vi "PmodACLOpen.vi"(7 "I2C Channel (0)":u8, 8 "Error In":errorcluster, 9 "Resolution":enum16{"2g", "4g", "8g", "16g"}(ring), 10 "ADXL345 Address":T1, 11 "LINX Resource":T2) -> (0 "Error Out":errorcluster, 1 "Resolution":enum16{"2g", "4g", "8g", "16g"}(ring), 3 "LINX Resource":T2)   [LabVIEW 2011, in "LMH-LINX.lvlib"]
doc: "Initialize the ADXL345 and bring it out of sleep mode."
uses:
  LMH-LINX.lvlib
  Private/Type Defs/LINX Ref.ctl
  Private/Type Defs/Platform.ctl
  Private/Type Defs/Interface.ctl
  Private/Device/Type Defs/LINX Device Config.ctl
  Private/Device/Type Defs/TCP Config.ctl
  Private/Device/Type Defs/Channels.ctl
  Accelerometer/ADXL345/Address.ctl
  Private/Device/Device.lvlib
  Accelerometer/ADXL345/ADXL345.lvlib
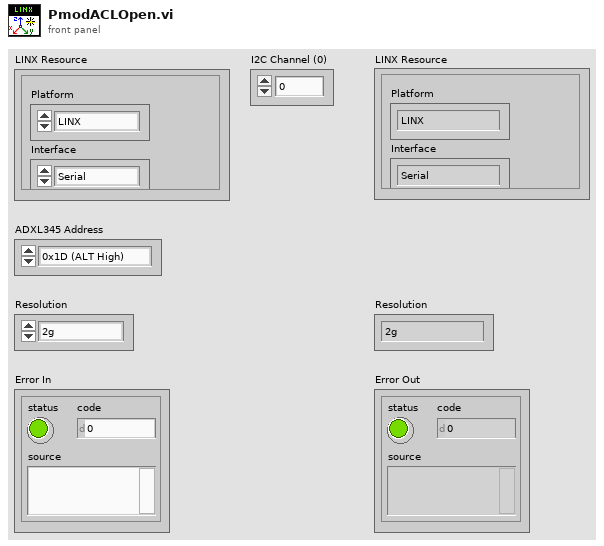
[diagram p1: front panel]
types:
  T1 = typedef "LMH-LINX.lvlib/ADXL345.lvlib/Address.ctl" = enum16{"0x1D (ALT High)", "0x53 (ALT Low)"}
  T2 = typedef "LMH-LINX.lvlib/LINX Ref.ctl" = cluster{"Platform":T3, "Interface":T4, "LINX Device Config":T5}
  T3 = typedef "LMH-LINX.lvlib/Platform.ctl" = enum16{"LINX", "myRIO"}
  T4 = typedef "LMH-LINX.lvlib/Interface.ctl" = enum16{"Serial", "TCP"}
  T5 = typedef "LMH-LINX.lvlib/Device.lvlib/LINX Device Config.ctl" = cluster{"Interface":T4, "COM Port":refnum<visa-resource-name>, "TCP Configuration":T6, "Device Family":u8, "Device ID":u8, "Device Name":string, "TCP Ref":refnum<k5>, "Channels":T7}
  T6 = typedef "LMH-LINX.lvlib/Device.lvlib/TCP Config.ctl" = cluster{"IP Address":string, "Port":u16}
  T7 = typedef "LMH-LINX.lvlib/Channels.ctl" = cluster{"DI":u8[], "DO":u8[], "AI":u8[], "AO":u8[], "PWM":u8[], "QE":u8[], "UART":u8[], "I2C 2":u8[], "SPI":u8[], "CAN":u8[], "Servo":u8[], "AI Ref (V)":dbl, "AO Ref (V)":dbl, "AO Resolution (Bits)":u8}
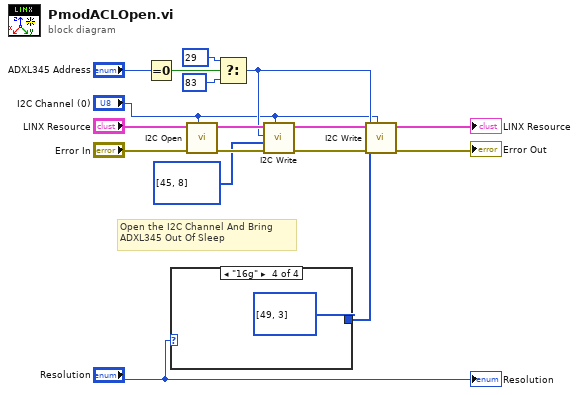
[diagram p0: block diagram]
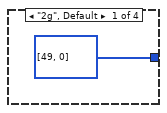
[diagram p2: hidden frame]
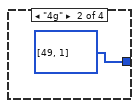
[diagram p3: hidden frame]
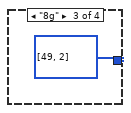
[diagram p4: hidden frame]
diagram:
  # "Open the I2C Channel And Bring \nADXL345 Out Of Sleep"
  n1 = Equal To 0?(x="ADXL345 Address") -> (x = 0?=w13:bool)
  n2 = case shown="\"16g\"" "Resolution" {
    tunnel: [u8[] [49, 0] ("Data") u8[] [49, 1] ("Data") u8[] [49, 2] ("Data") u8[] [49, 3] ("Data")] -> w7
    frame "2g", Default {
    }
    frame "4g" {
    }
    frame "8g" {
    }
    frame "16g" {
    }
  }
  n3 = call "I2C Open.vi"("I2C Channel (0)"="I2C Channel (0)", "Error In"="Error In", "LINX Resource"="LINX Resource") -> ("Error Out"=w16:errorcluster, "LINX Resource"=w17:T2)  [unwired: 7 in]
  n4 = Select(t=u8 29 ("I2C Slave Address (0)"), s=w13, f=u8 83 ("I2C Slave Address (0)")) -> (s? t:f=w2:u8)
  n5 = call "I2C Write.vi"("I2C Channel"="I2C Channel (0)", "Error In"=w16, "Data"=u8[] [45, 8], "I2C Slave Address (0)"=w2, "LINX Resource"=w17) -> ("Error Out"=w4:errorcluster, "LINX Resource"=w6:T2)  [unwired: 5 in]
  n6 = call "I2C Write.vi"("I2C Channel"="I2C Channel (0)", "Error In"=w4, "Data"=w7, "I2C Slave Address (0)"=w2, "LINX Resource"=w6) -> ("Error Out"=→"Error Out":errorcluster, "LINX Resource"=→"LINX Resource":T2)  [unwired: 5 in]
  "Resolution" <- "Resolution"
